vi "Photo Current.vi"(6 "T":dbl, 9 "k_i":dbl, 10 "I_sc":dbl, 11 "G":dbl) -> (3 "I_ph":dbl)   [LabVIEW 2024]
panel:
  in  "G 2":dbl
  in  "T 2":dbl
  # "-  298"
  # "="
  # "+"
  # "x"
  # "/ 1000"
  # "x"
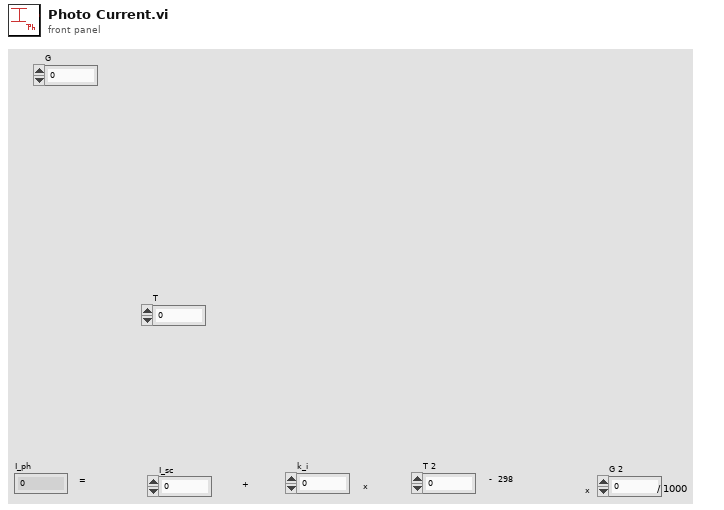
[diagram p1: front panel]
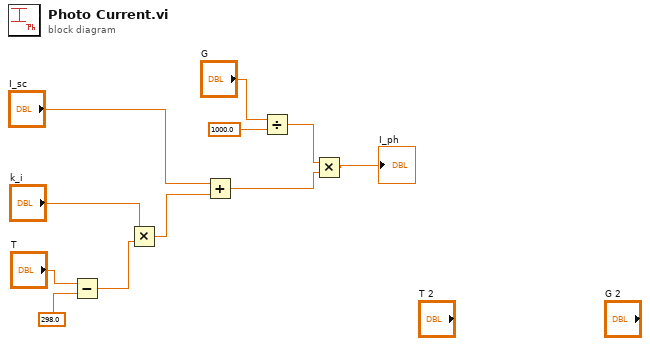
[diagram p0: block diagram]
diagram:
  n1 = Subtract(x="T", y=298.0) -> (x-y=w3:dbl)
  n2 = Multiply(x="k_i", y=w3) -> (x*y=w6:dbl)
  n3 = Add(x="I_sc", y=w6) -> (x+y=w10:dbl)
  n4 = Divide(x="G", y=1000.0) -> (x/y=w9:dbl)
  n5 = Multiply(x=w9, y=w10) -> (x*y=→"I_ph":dbl)
